vi "Act_shared_ELYs (SubVI).vi"(11 "output array in":sgl[][](array[numeric])) -> ()   [LabVIEW 2024]
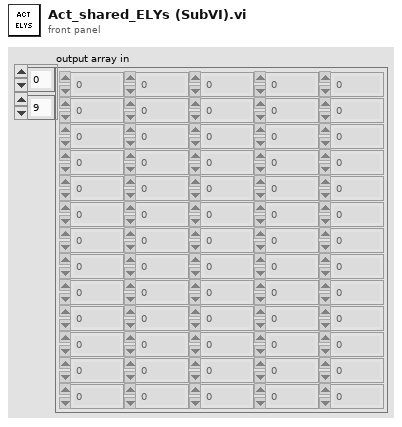
[diagram p1: front panel]
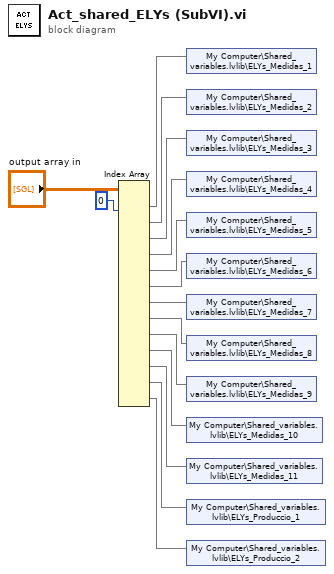
[diagram p0: block diagram]
diagram:
  n1 = Index Array(array="output array in", index (col) #1=0 ("disabled index (col)")) -> (element #1=w3:sgl[], element #2=w4:sgl[], element #3=w5:sgl[], element #4=w6:sgl[], element #5=w7:sgl[], element #6=w8:sgl[], element #7=w9:sgl[], element #8=w10:sgl[], element #9=w11:sgl[], element #10=w12:sgl[], element #11=w13:sgl[], element #12=w14:sgl[], element #13=w15:sgl[])  [unwired: 25 in]
  n2 = shared-variable "My Computer\\Shared_variables.lvlib\\ELYs_Medidas_1"(w3) -> ()  [unwired: 1 in, 1 out]
  n3 = shared-variable "My Computer\\Shared_variables.lvlib\\ELYs_Medidas_2"(w4) -> ()  [unwired: 1 in, 1 out]
  n4 = shared-variable "My Computer\\Shared_variables.lvlib\\ELYs_Medidas_3"(w5) -> ()  [unwired: 1 in, 1 out]
  n5 = shared-variable "My Computer\\Shared_variables.lvlib\\ELYs_Medidas_4"(w6) -> ()  [unwired: 1 in, 1 out]
  n6 = shared-variable "My Computer\\Shared_variables.lvlib\\ELYs_Medidas_5"(w7) -> ()  [unwired: 1 in, 1 out]
  n7 = shared-variable "My Computer\\Shared_variables.lvlib\\ELYs_Medidas_6"(w8) -> ()  [unwired: 1 in, 1 out]
  n8 = shared-variable "My Computer\\Shared_variables.lvlib\\ELYs_Medidas_7"(w9) -> ()  [unwired: 1 in, 1 out]
  n9 = shared-variable "My Computer\\Shared_variables.lvlib\\ELYs_Medidas_8"(w10) -> ()  [unwired: 1 in, 1 out]
  n10 = shared-variable "My Computer\\Shared_variables.lvlib\\ELYs_Medidas_9"(w11) -> ()  [unwired: 1 in, 1 out]
  n11 = shared-variable "My Computer\\Shared_variables.lvlib\\ELYs_Medidas_10"(w12) -> ()  [unwired: 1 in, 1 out]
  n12 = shared-variable "My Computer\\Shared_variables.lvlib\\ELYs_Medidas_11"(w13) -> ()  [unwired: 1 in, 1 out]
  n13 = shared-variable "My Computer\\Shared_variables.lvlib\\ELYs_Produccio_1"(w14) -> ()  [unwired: 1 in, 1 out]
  n14 = shared-variable "My Computer\\Shared_variables.lvlib\\ELYs_Produccio_2"(w15) -> ()  [unwired: 1 in, 1 out]
